vi "CreatePluginFromVI.vi"() -> ()   [LabVIEW 2020]
uses:
  <vilib>/Utility/miscctls.llb/LVPointTypeDef.ctl
  _Editor/MeasurementService Editor.lvlib
panel:
  out "error IO":errorcluster
  in  "vi path":path=path "C:/Users/rfriedma/Desktop/Sum.vi"
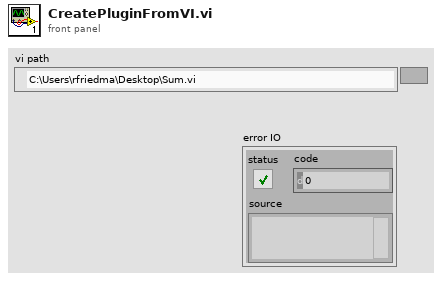
[diagram p1: front panel]
types:
  T1 = typedef "LVPointTypeDef.ctl" = cluster{"Horizontal":i16, "Vertical":i16}
  T2 = cluster{"ConfigurationUnbundle":refnum<vi>, "ResultsBundle":refnum<vi>}
  T3 = typedef "LVPositionTypeDef.ctl" = cluster{"Left":i32, "Top":i32}
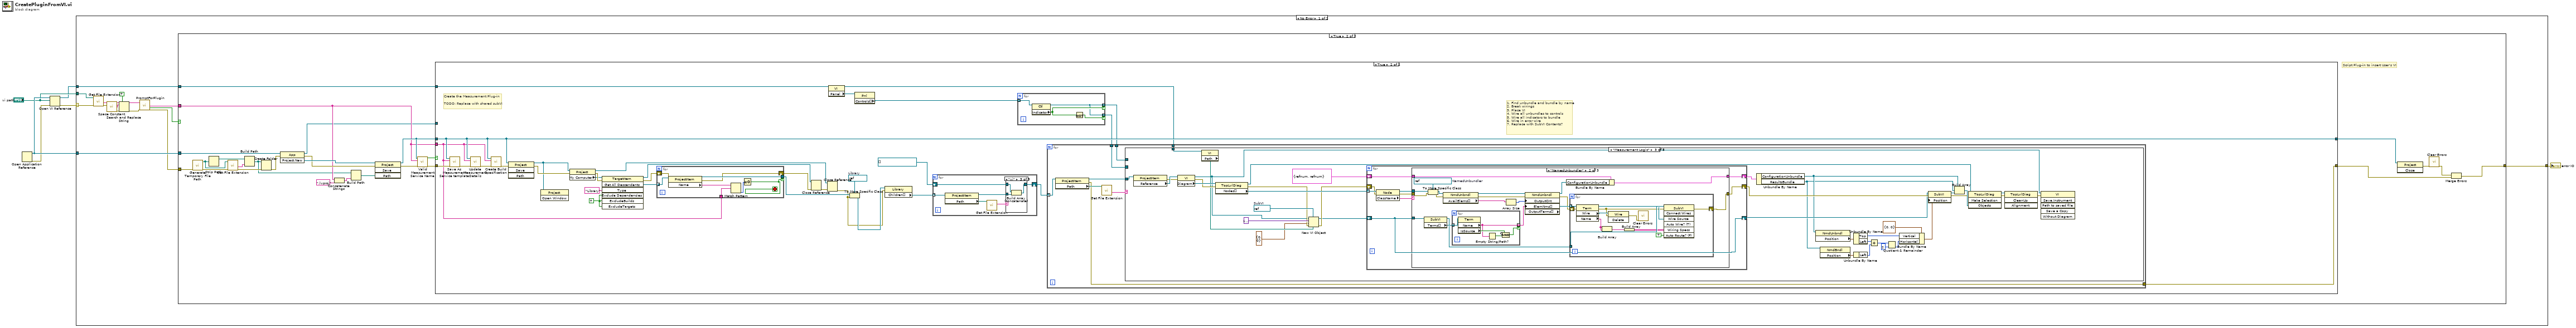
[diagram p0: block diagram]
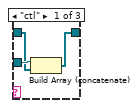
[diagram p4: hidden frame]
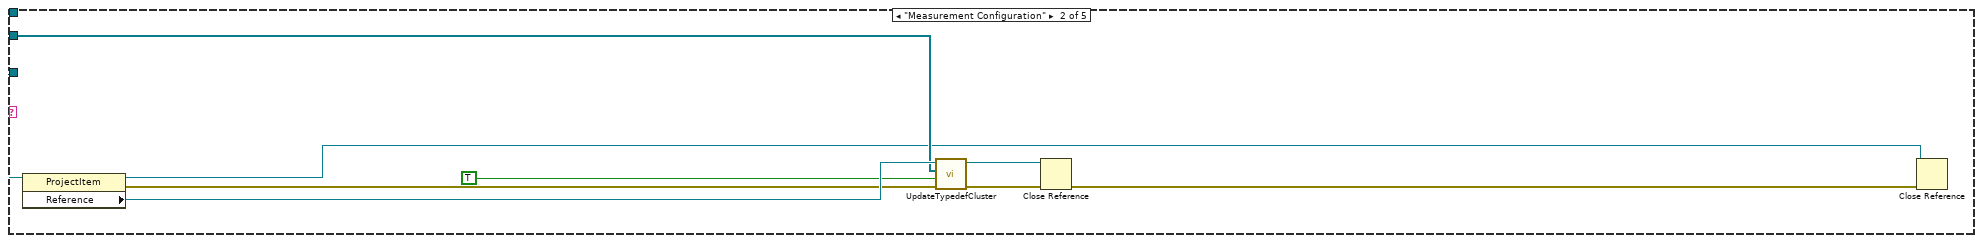
[diagram p7: hidden frame]
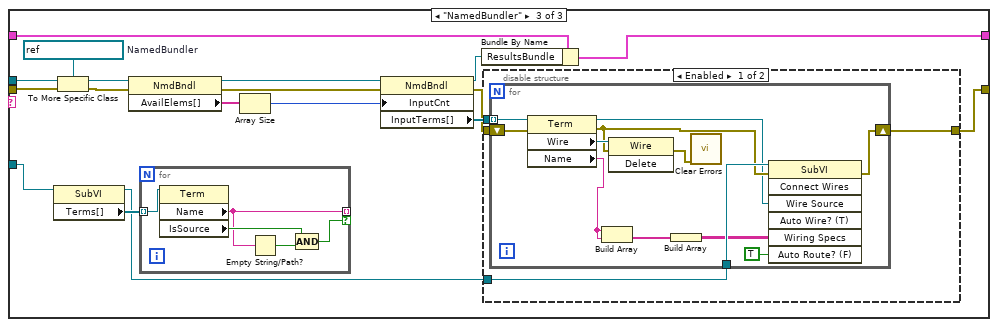
[diagram p9: hidden frame]
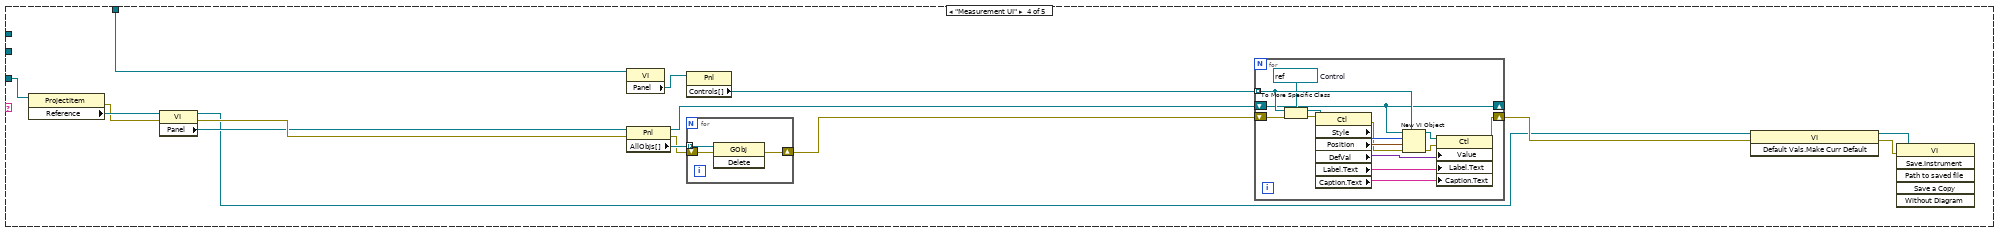
[diagram p11: hidden frame]
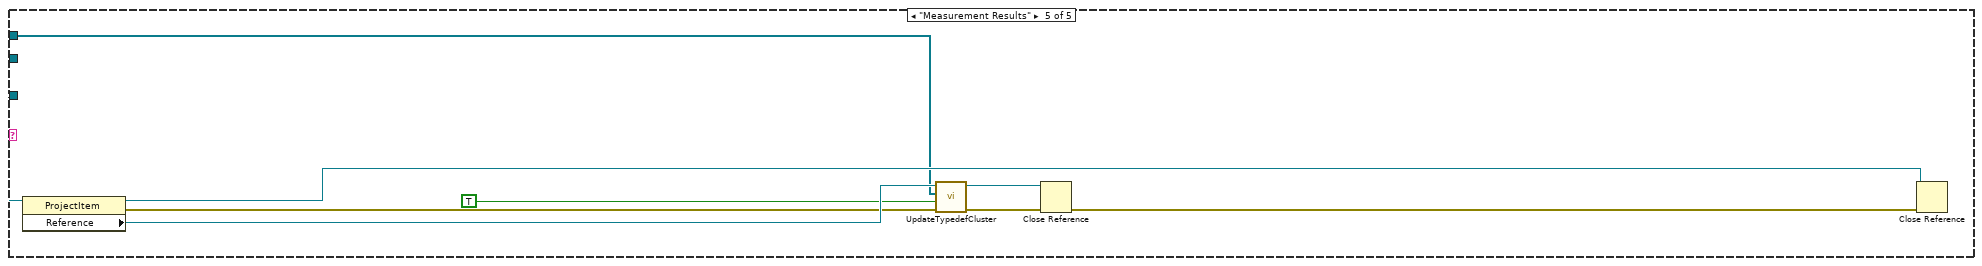
[diagram p12: hidden frame]
diagram:
  n1 = Open Application Reference() -> (0:w5:errorcluster, 3:w6:refnum<vi>)  [unwired: 4 in]
  n2 = Open VI Reference(application reference (local)=w6, vi path="vi path", error in (no error)=w5) -> (vi reference=w1:refnum<vi>, error out=w3:errorcluster)  [unwired: 3 in]
  n3 = case shown="No Error" w3 {
    selector: w3 -> [w11 w292]
    tunnel: w6 -> [w20 _]
    tunnel: "vi path" -> [w19 _]
    tunnel: [w12 w292] -> w2
    tunnel: w1 -> [w7 _]
    frame No Error {
      n4 = call <vilib>:"Get File Extension.vi"("error in (no error)"=w11, "file"=w19) -> ("error out"=w9:errorcluster, "filename without extension"=w18:string)  [unwired: 5 in, 3 out]
      n5 = call <vilib>:"Space Constant.vi"() -> ("String"=w17:string)
      n6 = Search and Replace String(replace all?=TRUE ("replace all? (F)"), input string=w18, search string=w17, error in=w9) -> (result string=w15:string, error out=w8:errorcluster)  [unwired: 4 in, 2 out]
      n7 = call "PromptForPlugin.vi"("Measurement Plug-in"=w15, "error in (no error)"=w8) -> ("Measurement Plug-in"=w13:string, "OK"=w14:bool, "error out"=w10:errorcluster)  [unwired: 15 in]
      n8 = case shown="True" w14 {
        tunnel: w20 -> [_ w42]
        tunnel: w10 -> [w21 w40]
        tunnel: w13 -> [_ w35]
        tunnel: [w21 w23] -> w12
        tunnel: w7 -> [_ w30]
        frame False {
        }
        frame True {
          # "Script Plug-in to insert User's VI"
          n9 = call <vilib>:"Generate Temporary File Path.vi"("error in (no error)"=w40) -> ("error out"=w44:errorcluster, "Unique Temporary File Path"=w43:path)  [unwired: 9 in]
          n10 = Strip Path(path=w43) -> (stripped path=w46:path)  [unwired: 1 out]
          n11 = call <vilib>:"Get File Extension.vi"("error in (no error)"=w44, "file"=w43) -> ("error out"=w32:errorcluster, "filename without extension"=w45:string)  [unwired: 5 in, 3 out]
          n12 = Build Path(base path=w46, name or relative path=w45) -> (appended path=w29:path)
          n13 = Create Folder(path (use dialog)=w29, error in=w32) -> (error out=w31:errorcluster)  [unwired: 1 in, 2 out]
          n14 = invoke class="App" method="Project.New"(reference=w42, error in=w31) -> (reference out=w28:refnum<vi>, error out=w41:errorcluster, "Project:New"=w47:refnum<vi>)  [unwired: 1 in]
          n15 = Concatenate Strings(w35, ".lvproj") -> (w34:string)
          n16 = Build Path(base path=w29, name or relative path=w34) -> (appended path=w22:path)
          n17 = invoke class="Project" method="Save"(reference=w47, error in=w41, "Path"=w22) -> (reference out=w38:refnum<vi>, error out=w37:errorcluster)  [unwired: 1 in, 2 out]
          n18 = call "Valid Measurement Service Name.vi"("error in"=w37, "Valid Service Name"=w35, "Project ref"=w38) -> ("error out"=w33:errorcluster, "Valid Name?"=w39:bool)  [unwired: 7 in]
          n19 = case shown="True" w39 {
            tunnel: w33 -> [w48 w81]
            tunnel: [w48 w55] -> w24
            tunnel: w38 -> [w49 w74]
            tunnel: w35 -> [_ w62]
            tunnel: w30 -> [_ w77]
            tunnel: w28 -> [_ _]
            tunnel: [w49 w74] -> w27
            frame False {
            }
            frame True {
              w61 = refnum<vi> refnum  # Library
              w67 = TRUE ("ExcludeDependencies")
              # "1. Find unbundle and bundle by name\n2. Break wirings\n3. Place VI\n4. Wire all unbundles to controls\n5. Wire all indicators to bundle\n6. Wire in error wire\n7. Replace with SubVI Contents?"
              # "Create the Measurement Plug-in\n\nTODO: Replace with shared subVI"
              n20 = call "Save As Measurement Service template.vi"("error in"=w81, "Measurement Service Name"=w62, "Project ref"=w74) -> ("error out"=w80:errorcluster)  [unwired: 8 in]
              n21 = call "Update Measurement Details.vi"("error in (no error)"=w80, "Measurement Service Name"=w62, "Project ref"=w74) -> ("error out"=w79:errorcluster)  [unwired: 8 in]
              n22 = call "Create Build Specification.vi"("error in (no error)"=w79, "Measurement Service Name"=w62, "Project in"=w74) -> ("error out"=w78:errorcluster)  [unwired: 8 in]
              n23 = invoke class="Project" method="Save"(reference=w74, error in=w78) -> (reference out=w54:refnum<vi>, error out=w63:errorcluster)  [unwired: 2 in, 2 out]
              n24 = invoke class="Project" method="Open Window"(reference=w54) -> ()  [unwired: 2 in, 3 out]
              n25 = property class="Project"(reference=w54, error in=w63) -> (reference out=w69:refnum<vi>, error out=w71:errorcluster, "My Computer"=w64:refnum<vi>)
              n26 = invoke class="TargetItem" method="Get All Descendents"(reference=w64, error in=w71, "Type"="Library", "Exclude Dependencies"=w67, "ExcludeBuilds"=w67, "ExcludeTargets"=w67) -> (reference out=w68:refnum<vi>, error out=w72:errorcluster, "All Descendents"=w66:refnum<vi>[])  [unwired: 1 in, 4 out]
              n27 = for {
                tunnel: w66 -> [w283] mode=indexing
                tunnel: w62 -> [w286]
                tunnel: [w281] -> w60 if=w284
                shift-right: [w280] -> w73
                shift-left: w72 -> [w282]
                stop <- w284 stop-if-true
                n28 = property class="ProjectItem"(reference=w283, error in=w282) -> (reference out=w281:refnum<vi>, error out=w280:errorcluster, "Name"=w287:string)
                n29 = Match Pattern(string=w287, regular expression=w286) -> (offset past match=w285:i32)  [unwired: 1 in, 3 out]
                n30 = Greater Or Equal To 0?(x=w285) -> (x >= 0?=w284:bool)
              }
              n31 = Close Reference(reference=w68, error in (no error)=w73) -> (error out=w70:errorcluster)
              n32 = Close Reference(reference=w69, error in (no error)=w70) -> (error out=w58:errorcluster)
              n33 = property class="VI"(reference=w77) -> (reference out=w50:refnum<vi>, "Panel"=w75:refnum<vi>)  [unwired: 1 in, 1 out]
              n34 = To More Specific Class(target class=w61, reference=w60, error in=w58) -> (specific class reference=w59:refnum<vi>)  [unwired: 1 out]
              n35 = property class="Pnl"(reference=w75) -> ("Controls[]"=w76:refnum<vi>[])  [unwired: 1 in, 2 out]
              n36 = property class="Library"(reference=w59, error in=w58) -> ("Children[]"=w52:refnum<vi>[])  [unwired: 2 out]
              n37 = for {
                tunnel: w52 -> [w87] mode=indexing
                shift-right: [w82] -> w51
                shift-left: refnum<vi>[] [] ("Array") -> [w83]
                n38 = property class="ProjectItem"(reference=w87) -> (reference out=w84:refnum<vi>, "Path"=w86:path)  [unwired: 1 in, 1 out]
                n39 = call <vilib>:"Get File Extension.vi"("file"=w86) -> ("lowercase file extension"=w85:string)  [unwired: 6 in, 4 out]
                n40 = case shown="\"vi\"" w85 {
                  tunnel: w84 -> [w90 _ w92]
                  tunnel: w83 -> [w89 w91 w93]
                  tunnel: [w88 w91 w94] -> w82
                  frame "ctl" {
                    n41 = Build Array (concatenate)(w90, w89) -> (w88:refnum<vi>[])
                  }
                  frame Default {
                  }
                  frame "vi" {
                    n42 = Build Array (concatenate)(w93, w92) -> (w94:refnum<vi>[])
                  }
                }
              }
              n43 = for {
                tunnel: w76 -> [w291] mode=indexing
                tunnel: [w289] -> w56 mode=indexing if=w290
                tunnel: [w289] -> w57 mode=indexing if=w288
                n44 = property class="Ctl"(reference=w291) -> (reference out=w289:refnum<vi>, "Indicator"=w290:bool)  [unwired: 1 in, 1 out]
                n45 = Not(x=w290) -> (.not. x?=w288:bool)
              }
              n46 = for {
                tunnel: w51 -> [w102] mode=indexing
                tunnel: w57 -> [w98]
                tunnel: w56 -> [w96]
                tunnel: [w97] -> w55
                tunnel: w50 -> [w95]
                n47 = property class="ProjectItem"(reference=w102) -> (reference out=w99:refnum<vi>, error out=w97:errorcluster, "Path"=w101:path)  [unwired: 1 in]
                n48 = call <vilib>:"Get File Extension.vi"("file"=w101) -> ("filename without extension"=w100:string)  [unwired: 6 in, 4 out]
                n49 = case shown="\"Measurement Logic\"" w100 {
                  tunnel: w99 -> [_ w111 w147 w252 w279]
                  tunnel: w98 -> [_ w108 _ _ _]
                  tunnel: w96 -> [_ _ _ _ w272]
                  tunnel: w95 -> [_ _ w143 w237 _]
                  frame Default {
                  }
                  frame "Measurement Configuration" {
                    n50 = property class="ProjectItem"(reference=w111) -> (reference out=w107:refnum<vi>, error out=w109:errorcluster, "Reference"=w110:refnum<vi>)  [unwired: 1 in]
                    n51 = call "UpdateTypedefCluster.vi"("error in (no error)"=w109, "Delete Existing Controls"=TRUE, "Control Refnums To Insert"=w108, "Typedef Cluster"=w110) -> ("error out"=w105:errorcluster, "Typedef Cluster out"=w106:refnum<vi>)  [unwired: 6 in]
                    n52 = Close Reference(reference=w106, error in (no error)=w105) -> (error out=w104:errorcluster)
                    n53 = Close Reference(reference=w107, error in (no error)=w104) -> ()  [unwired: 1 out]
                  }
                  frame "Measurement Logic" {
                    w128 = refnum<vi> refnum  # SubVI
                    n54 = property class="ProjectItem"(reference=w147) -> (error out=w145:errorcluster, "Reference"=w146:refnum<vi>)  [unwired: 1 in, 1 out]
                    n55 = property class="VI"(reference=w146, error in=w145) -> (reference out=w121:refnum<vi>, error out=w144:errorcluster, "Diagram"=w149:refnum<vi>)
                    n56 = property class="VI"(reference=w143) -> ("Path"=w127:path)  [unwired: 1 in, 2 out]
                    n57 = property class="TopLvlDiag"(reference=w149, error in=w144) -> (reference out=w120:refnum<vi>, error out=w126:errorcluster, "Nodes[]"=w148:refnum<vi>[])
                    n58 = New VI Object(vi object class=w128, owner refnum=w121, style=variant, position/next to=T1 {"Horizontal"=0, "Vertical"=0} ("location"), 6:w127, 8:w126) -> (object refnum=w123:refnum<vi>, 0:w125:errorcluster)  [unwired: 2 in]
                    n59 = for {
                      tunnel: w148 -> [w158] mode=indexing
                      shift-right: [w153] -> w130
                      shift-left: w125 -> [w155]
                      shift-right: [w151] -> w141
                      shift-left: T2 {"ConfigurationUnbundle"=refnum, "ResultsBundle"=refnum} -> [w152]
                      shift-right: [w150] -> w122
                      shift-left: w123 -> [w150]
                      n60 = property class="Node"(reference=w158, error in=w155) -> (reference out=w156:refnum<vi>, error out=w154:errorcluster, "ClassName"=w157:string)
                      n61 = case shown="\"NamedUnbundler\"" w157 {
                        tunnel: w156 -> [_ w179 w214]
                        tunnel: w154 -> [w160 w175 w212]
                        tunnel: [w160 w167 w200] -> w153
                        tunnel: w152 -> [w159 w170 w211]
                        tunnel: [w159 w171 w210] -> w151
                        tunnel: w150 -> [_ w166 w198]
                        frame Default {
                        }
                        frame "NamedUnbundler" {
                          w178 = refnum<vi> refnum  # NamedUnbundler
                          n62 = property class="SubVI"(reference=w166) -> (reference out=w161:refnum<vi>, "Terms[]"=w165:refnum<vi>[])  [unwired: 1 in, 1 out]
                          n63 = To More Specific Class(target class=w178, reference=w179, error in=w175) -> (specific class reference=w177:refnum<vi>, error out=w174:errorcluster)
                          n64 = property class="NmdUnbndl"(reference=w177, error in=w174) -> (reference out=w176:refnum<vi>, error out=w173:errorcluster, "AvailElems[]"=w162:string[])
                          n65 = for {
                            tunnel: w165 -> [w196] mode=indexing
                            tunnel: [w193] -> w163 mode=indexing if=w194
                            n66 = property class="Term"(reference=w196) -> ("Name"=w193:string, "IsSource"=w195:bool)  [unwired: 1 in, 2 out]
                            n67 = Empty String/Path?(string/path=w193) -> (empty?=w192:bool)
                            n68 = Compound Arithmetic op=AND(invert w195, w192) -> (w194:bool)
                          }
                          n69 = Array Size(array=w162) -> (size(s)=w164:i32)
                          n70 = property class="NmdUnbndl"(reference=w176, error in=w173, "OutputCnt"=w164, "ElemNms[]"=w163) -> (reference out=w172:refnum<vi>, error out=w168:errorcluster, "OutputTerms[]"=w169:refnum<vi>[])
                          n71 = Bundle By Name(cluster=w170, "ConfigurationUnbundle"=w172) -> (w171:T2)
                          n72 = for {
                            tunnel: w169 -> [w191] mode=indexing
                            shift-right: [w181] -> w167
                            shift-left: w168 -> [w189]
                            tunnel: w161 -> [w187]
                            n73 = property class="Term"(reference=w191, error in=w189) -> (reference out=w186:refnum<vi>, error out=w182:errorcluster, "Wire"=w190:refnum<vi>, "Name"=w185:string)
                            n74 = Build Array(w185, w185) -> (w184:string[])
                            n75 = invoke class="Wire" method="Delete"(reference=w190, error in=w182) -> (error out=w188:errorcluster)  [unwired: 1 in, 2 out]
                            n76 = Build Array(w184) -> (w183:string[][])
                            n77 = call <vilib>:"Clear Errors.vi"("error in (no error)"=w188) -> ()  [unwired: 5 in, 2 out]
                            n78 = invoke class="SubVI" method="Connect Wires"(reference=w187, error in=w182, "Wire Source"=w186, "Wiring Specs"=w183, "Auto Route? (F)"=TRUE) -> (error out=w181:errorcluster)  [unwired: 2 in, 6 out]
                          }
                        }
                        frame "NamedBundler" {
                          w213 = refnum<vi> refnum  # NamedBundler
                          n79 = property class="SubVI"(reference=w198) -> (reference out=w197:refnum<vi>, "Terms[]"=w199:refnum<vi>[])  [unwired: 1 in, 1 out]
                          n80 = To More Specific Class(target class=w213, reference=w214, error in=w212) -> (specific class reference=w204:refnum<vi>, error out=w205:errorcluster)
                          n81 = property class="NmdBndl"(reference=w204, error in=w205) -> (reference out=w209:refnum<vi>, error out=w207:errorcluster, "AvailElems[]"=w208:string[])
                          n82 = for {
                            tunnel: w199 -> [w219] mode=indexing
                            tunnel: [w216] -> _ mode=indexing if=w217
                            n83 = property class="Term"(reference=w219) -> ("Name"=w216:string, "IsSource"=w218:bool)  [unwired: 1 in, 2 out]
                            n84 = Empty String/Path?(string/path=w216) -> (empty?=w215:bool)
                            n85 = Compound Arithmetic op=AND(w218, w215) -> (w217:bool)
                          }
                          n86 = Array Size(array=w208) -> (size(s)=w206:i32)
                          n87 = property class="NmdBndl"(reference=w209, error in=w207, "InputCnt"=w206) -> (reference out=w203:refnum<vi>, error out=w201:errorcluster, "InputTerms[]"=w202:refnum<vi>[])
                          n88 = Bundle By Name(cluster=w211, "ResultsBundle"=w203) -> (w210:T2)
                          n89 = disable-structure shown="Enabled" {
                            disable-tunnel: w202 -> [w223 _]
                            disable-tunnel: w201 -> [w222 w236]
                            disable-tunnel: [w221 w236] -> w200
                            disable-tunnel: w197 -> [w220 _]
                            frame Enabled {
                              n90 = for {
                                tunnel: w223 -> [w235] mode=indexing
                                shift-right: [w228] -> w221
                                shift-left: w222 -> [w233]
                                tunnel: w220 -> [w230]
                                n91 = property class="Term"(reference=w235, error in=w233) -> (reference out=w227:refnum<vi>, error out=w229:errorcluster, "Wire"=w234:refnum<vi>, "Name"=w226:string)
                                n92 = Build Array(w226, w226) -> (w231:string[])
                                n93 = invoke class="Wire" method="Delete"(reference=w234, error in=w229) -> (error out=w232:errorcluster)  [unwired: 1 in, 2 out]
                                n94 = Build Array(w231) -> (w225:string[][])
                                n95 = call <vilib>:"Clear Errors.vi"("error in (no error)"=w232) -> ()  [unwired: 5 in, 2 out]
                                n96 = invoke class="SubVI" method="Connect Wires"(reference=w230, error in=w229, "Wire Source"=w227, "Wiring Specs"=w225, "Auto Route? (F)"=TRUE) -> (error out=w228:errorcluster)  [unwired: 2 in, 6 out]
                              }
                            }
                            frame Disabled {
                            }
                          }
                        }
                      }
                    }
                    n97 = Unbundle By Name(w141) -> ("ConfigurationUnbundle"=w119:refnum<vi>, "ResultsBundle"=w118:refnum<vi>)
                    n98 = property class="NmdUnbndl"(reference=w119) -> ("Position"=w140:T3)  [unwired: 1 in, 2 out]
                    n99 = property class="NmdBndl"(reference=w118) -> ("Position"=w139:T3)  [unwired: 1 in, 2 out]
                    n100 = Unbundle By Name(w140) -> ("Top"=w137:i32, "Left"=w135:i32)
                    n101 = Unbundle By Name(w139) -> ("Left"=w136:i32)
                    n102 = Add(x=w135, y=w136) -> (x+y=w134:i32)
                    n103 = Quotient & Remainder(x=w134, y=2) -> (floor(x/y)=w132:i32)  [unwired: 1 out]
                    n104 = Bundle By Name(cluster=T1 {"Horizontal"=0, "Vertical"=0} ("location"), "Vertical"=w137, "Horizontal"=w132) -> (w131:T1)
                    n105 = property class="SubVI"(reference=w122, error in=w130, "Position"=w131) -> (reference out=w117:refnum<vi>, error out=w114:errorcluster)
                    n106 = Build Array(w119, w118, w117) -> (w116:refnum<vi>[])
                    n107 = invoke class="TopLvlDiag" method="Make Selection"(reference=w120, error in=w114, "Objects"=w116) -> (reference out=w115:refnum<vi>, error out=w113:errorcluster)  [unwired: 1 in, 2 out]
                    n108 = invoke class="TopLvlDiag" method="CleanUp"(reference=w115, error in=w113) -> (error out=w112:errorcluster)  [unwired: 2 in, 3 out]
                    n109 = invoke class="VI" method="Save.Instrument"(reference=w121, error in=w112) -> ()  [unwired: 4 in, 6 out]
                  }
                  frame "Measurement UI" {
                    n110 = property class="ProjectItem"(reference=w252) -> (error out=w246:errorcluster, "Reference"=w251:refnum<vi>)  [unwired: 1 in, 1 out]
                    n111 = property class="VI"(reference=w251, error in=w246) -> (reference out=w238:refnum<vi>, error out=w245:errorcluster, "Panel"=w239:refnum<vi>)
                    n112 = property class="VI"(reference=w237) -> ("Panel"=w249:refnum<vi>)  [unwired: 1 in, 2 out]
                    n113 = property class="Pnl"(reference=w239, error in=w245) -> (reference out=w248:refnum<vi>, error out=w244:errorcluster, "AllObjs[]"=w250:refnum<vi>[])
                    n114 = property class="Pnl"(reference=w249) -> ("Controls[]"=w247:refnum<vi>[])  [unwired: 1 in, 2 out]
                    n115 = for {
                      tunnel: w250 -> [w270] mode=indexing
                      shift-right: [w268] -> w243
                      shift-left: w244 -> [w269]
                      n116 = invoke class="GObj" method="Delete"(reference=w270, error in=w269) -> (error out=w268:errorcluster)  [unwired: 1 in, 2 out]
                    }
                    n117 = for {
                      tunnel: w247 -> [w267] mode=indexing
                      shift-right: [w262] -> _
                      shift-left: w248 -> [w262]
                      shift-right: [w255] -> w242
                      shift-left: w243 -> [w259]
                      w266 = refnum<vi> refnum  # Control
                      n118 = To More Specific Class(target class=w266, reference=w267, error in=w259) -> (specific class reference=w265:refnum<vi>, error out=w258:errorcluster)
                      n119 = property class="Ctl"(reference=w265, error in=w258) -> (error out=w257:errorcluster, "Style"=w264:u32, "Position"=w263:T3, "DefVal"=w260:variant, "Label.Text"=w254:string, "Caption.Text"=w253:string)  [unwired: 1 out]
                      n120 = New VI Object(vi object class=w267, owner refnum=w262, style=w264, position/next to=w263, 8:w257) -> (object refnum=w261:refnum<vi>, 0:w256:errorcluster)  [unwired: 3 in]
                      n121 = property class="Ctl"(reference=w261, error in=w256, "Value"=w260, "Label.Text"=w254, "Caption.Text"=w253) -> (error out=w255:errorcluster)  [unwired: 1 out]
                    }
                    n122 = invoke class="VI" method="Default Vals.Make Curr Default"(reference=w238, error in=w242) -> (reference out=w241:refnum<vi>, error out=w240:errorcluster)  [unwired: 1 in, 1 out]
                    n123 = invoke class="VI" method="Save.Instrument"(reference=w241, error in=w240) -> ()  [unwired: 4 in, 6 out]
                  }
                  frame "Measurement Results" {
                    n124 = property class="ProjectItem"(reference=w279) -> (reference out=w276:refnum<vi>, error out=w277:errorcluster, "Reference"=w278:refnum<vi>)  [unwired: 1 in]
                    n125 = call "UpdateTypedefCluster.vi"("error in (no error)"=w277, "Delete Existing Controls"=TRUE, "Control Refnums To Insert"=w272, "Typedef Cluster"=w278) -> ("error out"=w274:errorcluster, "Typedef Cluster out"=w275:refnum<vi>)  [unwired: 6 in]
                    n126 = Close Reference(reference=w275, error in (no error)=w274) -> (error out=w273:errorcluster)
                    n127 = Close Reference(reference=w276, error in (no error)=w273) -> ()  [unwired: 1 out]
                  }
                }
              }
            }
          }
          n128 = invoke class="Project" method="Close"(reference=w27) -> (error out=w26:errorcluster)  [unwired: 2 in, 2 out]
          n129 = call <vilib>:"Clear Errors.vi"("error in (no error)"=w26) -> ("error out"=w25:errorcluster)  [unwired: 5 in, 1 out]
          n130 = Merge Errors(w25, w24) -> (w23:errorcluster)
        }
      }
    }
    frame Error {
    }
  }
  "error IO" <- w2
